vi "Butterfly_PullDown RC no data.vi"(0 "Semiconductor Module Context":T1, 1 "RFPins":string[](array[string]), 2 "current level":dbl=0.01 format="%_6p", 5 "error in (no error)":errorcluster, 7 "Start_v":dbl=10.0 format="%#_13g", 9 "Stop_v":dbl=41.0 format="%#_13g", 11 "Step_v":dbl=1.0) -> (14 "Semiconductor Module Context Out":T1, 19 "error out":errorcluster)   [LabVIEW 2013]
uses:
  <vilib>/NI_TestStand_SemiconductorModule/NI_TestStand_Semiconductor_Module.lvlibp/PinMap/General/SemiconductorModuleContext.ctl
  <instrlib>/niDCPower/nidcpower.llb/niDCPower Wait For Event - Event.ctl
  <vilib>/NI_TestStand_SemiconductorModule/NI_TestStand_Semiconductor_Module.lvlibp/PinMap/DC Power/PinsToNIDCPowerSessions.vi
  <vilib>/NI_TestStand_SemiconductorModule/NI_TestStand_Semiconductor_Module.lvlibp
panel:
  out "step":i32
  out "Instrument Session":refnum<k15>
  out "sites and pins loop iter":i32
  out "Channel List":string
  out "BF values":dbl[](array[numeric])
  out "BF Names":string[](array[string])
  out "R Array":dbl[](array[numeric])
  out "BFSamples":i32
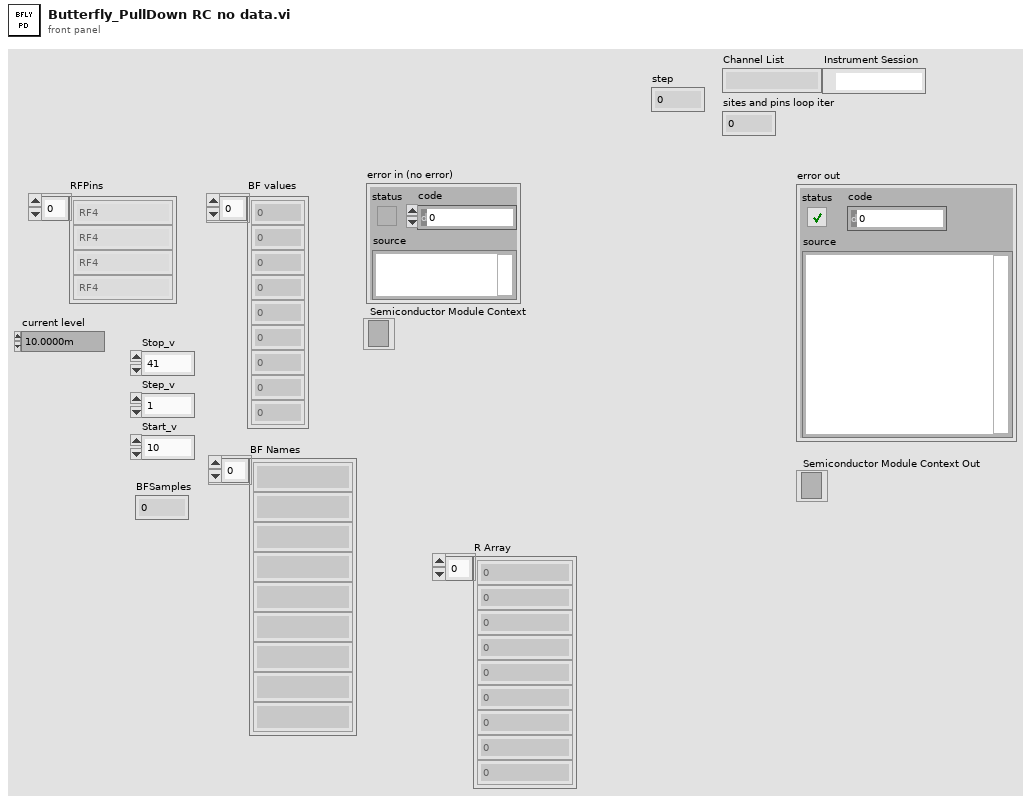
[diagram p1: front panel]
types:
  T1 = typedef "NI_TestStand_Semiconductor_Module.lvlibp/SemiconductorModuleContext.ctl" = refnum<k7>
  T2 = typedef "niDCPower Wait For Event - Event.ctl" = i32
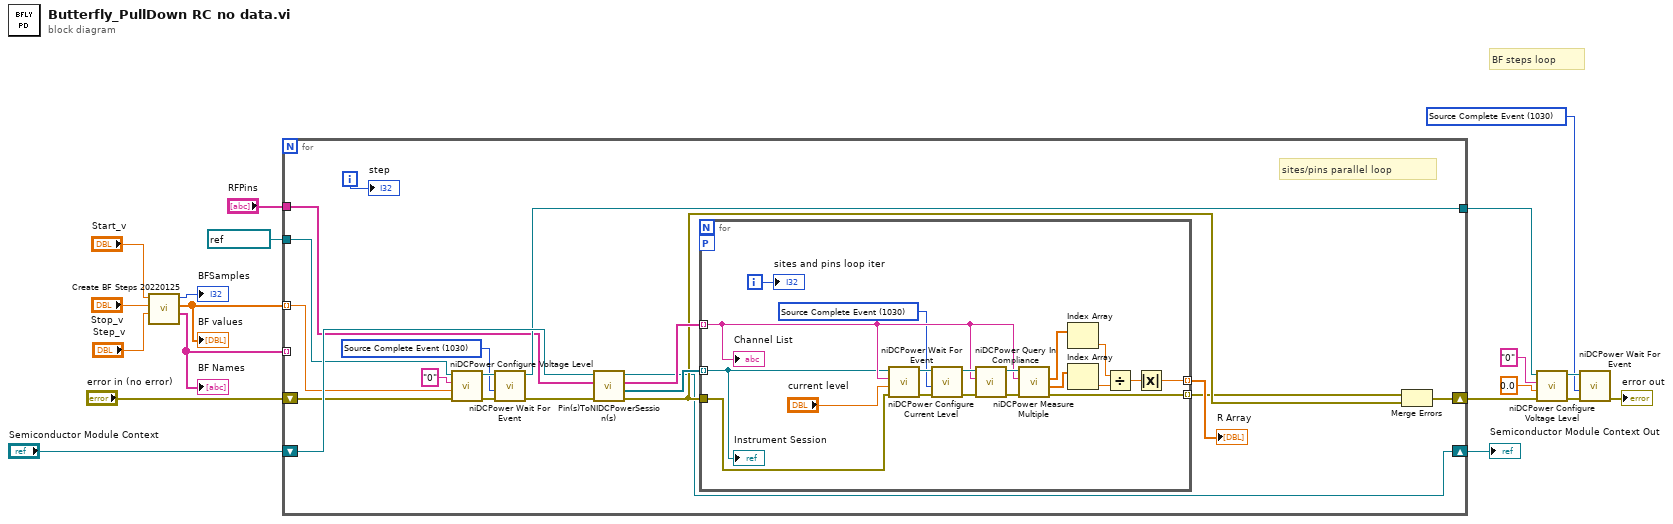
[diagram p0: block diagram]
diagram:
  w7 = T2 1030 items=["Source Complete Event"=1030, "Measure Complete Event"=1031, "Sequence Iteration Complete Event"=1032, "Sequence Engine Done Event"=1033, "Pulse Complete Event"=1051, "Ready For Pulse Trigger Event"=1052] ("event")
  # "BF steps loop"
  n1 = call "Create BF Steps 20220125.vi"("Step_v"="Step_v", "Stop_v"="Stop_v", "Start_v"="Start_v") -> ("BF Names"=w5:string[], "BF values"=w4:dbl[], "BFSamples"=→"BFSamples":i32)  [unwired: 6 in]
  "BF Names" <- w5
  "BF values" <- w4
  n2 = for {
    shift-right: [w20] -> w1
    shift-left: "error in (no error)" -> [w34]
    tunnel: w4 -> [w32] mode=indexing
    tunnel: refnum<k15> "4139_1" ("instrument handle") -> [w31]
    tunnel: [w30] -> w11
    tunnel: "RFPins" -> [w26]
    tunnel: w5 -> [_] mode=indexing
    shift-right: [w21] -> w2
    shift-left: "Semiconductor Module Context" -> [w38]
    i -> [w27]
    w36 = T2 1030 items=["Source Complete Event"=1030, "Measure Complete Event"=1031, "Sequence Iteration Complete Event"=1032, "Sequence Engine Done Event"=1033, "Pulse Complete Event"=1051, "Ready For Pulse Trigger Event"=1052] ("event")
    # "sites/pins parallel loop"
    n3 = call <instrlib>:"niDCPower Configure Voltage Level.vi"("error in (no error)"=w34, "voltage level"=w32, "channel name"="0", "instrument handle"=w31) -> ("error out"=w35:errorcluster, "instrument handle out"=w37:refnum<k15>)  [unwired: 6 in]
    n4 = call <instrlib>:"niDCPower Wait For Event.vi"("error in (no error)"=w35, "event"=w36, "instrument handle"=w37) -> ("error out"=w33:errorcluster, "instrument handle out"=w30:refnum<k15>)  [unwired: 7 in]
    n5 = call-poly <vilib>:"Pin(s)ToNIDCPowerSession(s).vi"("error in (no error)"=w33, "Pins"=w26, "Semiconductor Module Context"=w38) -> ("error out"=w23:errorcluster, "Instrument Sessions"=w29:refnum<k15>[], "Channel Lists"=w28:string[], "Semiconductor Module Context Out"=w21:T1)  [unwired: 4 in, 1 out]
    n6 = for {
      tunnel: w28 -> [w44] mode=indexing
      tunnel: w29 -> [w41] mode=indexing
      tunnel: w23 -> [w42]
      tunnel: [w45] -> w25 mode=indexing
      tunnel: [w39] -> w22 mode=indexing
      workers-P: _ -> [_]
      i -> [w40]
      w43 = T2 1030 items=["Source Complete Event"=1030, "Measure Complete Event"=1031, "Sequence Iteration Complete Event"=1032, "Sequence Engine Done Event"=1033, "Pulse Complete Event"=1051, "Ready For Pulse Trigger Event"=1052] ("event")
      n7 = call <instrlib>:"niDCPower Configure Current Level.vi"("error in (no error)"=w42, "current level"="current level", "channel name"=w44, "instrument handle"=w41) -> ("error out"=w53:errorcluster, "instrument handle out"=w52:refnum<k15>)  [unwired: 6 in]
      n8 = call <instrlib>:"niDCPower Wait For Event.vi"("error in (no error)"=w53, "event"=w43, "instrument handle"=w52) -> ("error out"=w57:errorcluster, "instrument handle out"=w56:refnum<k15>)  [unwired: 7 in]
      n9 = call <instrlib>:"niDCPower Query In Compliance.vi"("error in (no error)"=w57, "channel name"=w44, "instrument handle"=w56) -> ("error out"=w54:errorcluster, "instrument handle out"=w55:refnum<k15>)  [unwired: 6 in, 1 out]
      n10 = call <instrlib>:"niDCPower Measure Multiple.vi"("error in (no error)"=w54, "channel name"=w44, "instrument handle"=w55) -> ("error out"=w39:errorcluster, "current measurements"=w46:dbl[], "voltage measurements"=w47:dbl[])  [unwired: 5 in, 1 out]
      n11 = Index Array(array=w47) -> (element=w49:dbl)  [unwired: 1 in]
      n12 = Index Array(array=w46) -> (element=w48:dbl)  [unwired: 1 in]
      n13 = Divide(x=w49, y=w48) -> (x/y=w50:dbl)
      n14 = Absolute Value(x=w50) -> (abs(x)=w45:dbl)
      "Channel List" <- w44
      "sites and pins loop iter" <- w40
      "Instrument Session" <- w41
    }
    "R Array" <- w25
    n15 = Merge Errors(w22, w23) -> (w20:errorcluster)
    "step" <- w27
  }
  "Semiconductor Module Context Out" <- w2
  n16 = call <instrlib>:"niDCPower Configure Voltage Level.vi"("error in (no error)"=w1, "voltage level"=0.0, "channel name"="0", "instrument handle"=w11) -> ("error out"=w10:errorcluster, "instrument handle out"=w8:refnum<k15>)  [unwired: 6 in]
  n17 = call <instrlib>:"niDCPower Wait For Event.vi"("error in (no error)"=w10, "event"=w7, "instrument handle"=w8) -> ("error out"=→"error out":errorcluster)  [unwired: 7 in, 1 out]
